vi "Update Build Versions.vi"(8 "error in (no error)":errorcluster, 9 "Product Name":string, 10 "Package Version":string, 11 "Package Source Folder":path) -> (0 "error out":errorcluster)   [LabVIEW 2016]
uses:
  <vilib>/AppBuilder/AB_API_Simple/Build Specification Version.ctl
  <vilib>/AppBuilder/AB_API_Simple/Set Build Specification Version (path).vi
  <vilib>/AppBuilder/AB_API_Simple/NI_App_Builder_API.lvlib
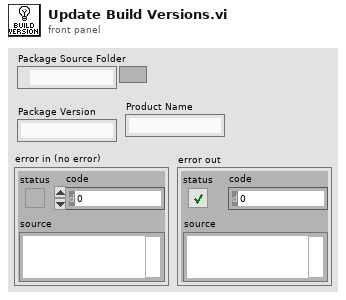
[diagram p1: front panel]
types:
  T1 = typedef "NI_App_Builder_API.lvlib/Build Specification Version.ctl" = cluster{"Major":u16, "Minor":u16, "Fix":u16, "Build":u16}
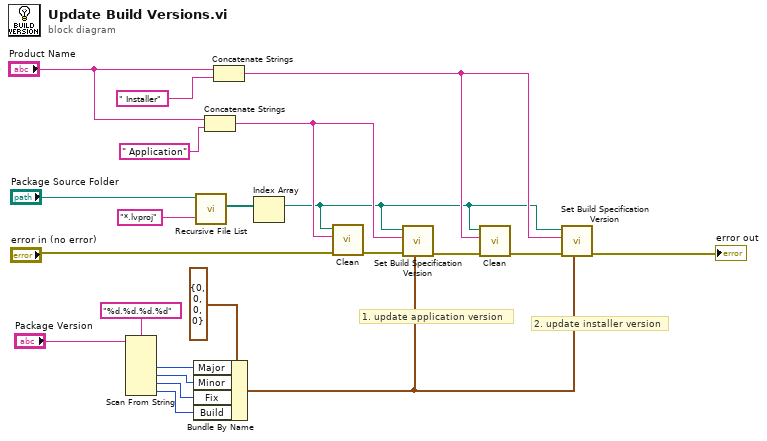
[diagram p0: block diagram]
diagram:
  # "2. update installer version"
  # "1. update application version"
  n1 = Scan From String(format string="%d.%d.%d.%d", input string="Package Version") -> (output 1=w16:i32, output 2=w19:i32, output 3=w15:i32, output 4=w18:i32)  [unwired: 6 in, 3 out]
  n2 = Bundle By Name(cluster=T1 {"Major"=0, "Minor"=0, "Fix"=0, "Build"=0} ("Build Specification Version"), "Major"=w16, "Minor"=w19, "Fix"=w15, "Build"=w18) -> (w20:T1)
  n3 = call <vilib>:"Recursive File List.vi"("pattern"="*.lvproj", "Folder Path"="Package Source Folder") -> ("All Files in Dir"=w2:path[])  [unwired: 5 in, 4 out]
  n4 = Concatenate Strings("Product Name", " Application" ("Name of target (My Computer)")) -> (w8:string)
  n5 = Concatenate Strings("Product Name", " Installer" ("Name of target (My Computer)")) -> (w6:string)
  n6 = Index Array(array=w2) -> (element=w1:path)  [unwired: 1 in]
  n7 = call <vilib>:"Clean.vi"("error in (no error)"="error in (no error)", "Name of build specification (if empty: clean all)"=w8, "Path to project"=w1) -> ("error out"=w13:errorcluster)  [unwired: 8 in]
  n8 = call-poly <vilib>:"Set Build Specification Version.vi"("Build Specification Version"=w20, "error in (no error)"=w13, "Name of build specification"=w8, "Path to project"=w1) -> ("error out"=w12:errorcluster)  [unwired: 7 in]
  n9 = call <vilib>:"Clean.vi"("error in (no error)"=w12, "Name of build specification (if empty: clean all)"=w6, "Path to project"=w1) -> ("error out"=w11:errorcluster)  [unwired: 8 in]
  n10 = call-poly <vilib>:"Set Build Specification Version.vi"("Build Specification Version"=w20, "error in (no error)"=w11, "Name of build specification"=w6, "Path to project"=w1) -> ("error out"=→"error out":errorcluster)  [unwired: 7 in]
